vi "Report Error.vi"(8 "error in (no error)":errorcluster, 9 "Message":string, 10 "Context":string, 11 "VolatusAPI in":refnum<class "VolatusAPI.lvclass">) -> (0 "error out":errorcluster, 3 "VolatusAPI out":refnum<class "VolatusAPI.lvclass">)   [LabVIEW 2020, in "Volatus.lvlib" / "VolatusAPI.lvclass"]
uses:
  VolatusAPI.lvclass
  Event.ctl
  Event Level.ctl
  VolatusAPI.lvclass/VolatusAPI.ctl
  MessageQ/MessageQ.lvclass/MessageQ.ctl
  Volatus.lvlib
  MessageQ/MessageQ.lvclass
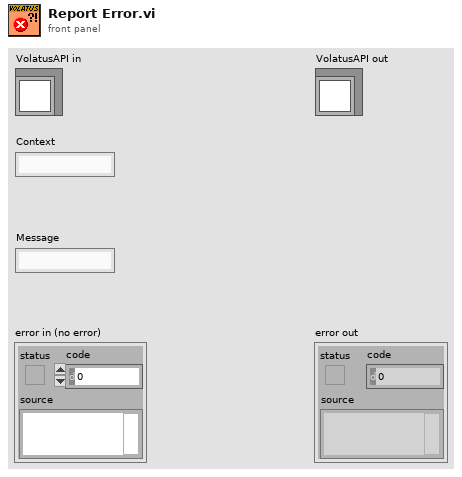
[diagram p1: front panel]
types:
  T1 = typedef "Volatus.lvlib/Event Level.ctl" = enum16{"Debug", "Info", "Warning", "Error"}
  T2 = typedef "Volatus.lvlib/Event.ctl" = cluster{"Time Stamp":timestamp, "Event Level":T1, "Context":string, "Message":string, "Error":errorcluster}
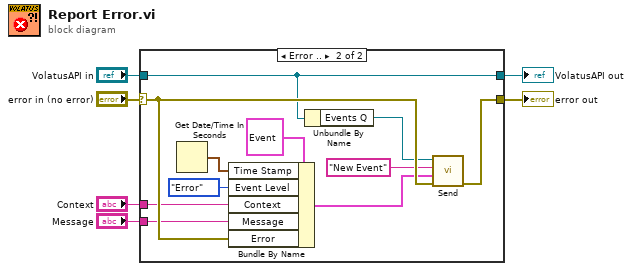
[diagram p0: block diagram]
diagram:
  n1 = case shown="Error .." "error in (no error)" {
    selector: "error in (no error)" -> [w7 w19]
    tunnel: "VolatusAPI in" -> [w8 w13]
    tunnel: [w8 w13] -> w4
    tunnel: [w7 w9] -> w3
    tunnel: "Context" -> [_ w15]
    tunnel: "Message" -> [_ w14]
    frame No Error {
    }
    frame Error {
      n2 = Get Date/Time In Seconds() -> (seconds since 1Jan1904=w16:timestamp)
      n3 = Bundle By Name(cluster=T2 {"Time Stamp"=timestamp(0 s since 1904-01-01), "Event Level"=enum."Info", "Context"="", "Message"="", "Error"={"status"=FALSE, "code"=0, "source"=""}} ("Event"), "Time Stamp"=w16, "Event Level"=Event_Level."Error", "Context"=w15, "Message"=w14, "Error"=w19) -> (w10:T2)
      n4 = Unbundle By Name(w13) -> ("Events Q"=w12:refnum<class "MessageQ.lvclass">)
      n5 = call "Send.vi"("error in (no error)"=w19, "Data"=w10, "ID"="New Event", "MessageQ in"=w12) -> ("error out"=w9:errorcluster)  [unwired: 6 in, 1 out]
    }
  }
  "error out" <- w3
  "VolatusAPI out" <- w4
